vi "Enable_disable State on Multiple Controls.vi"(8 "error in (no error)":errorcluster, 9 "Disabled":T1(ring)=enum."Disabled and Grayed Out", 10 "Disable control?":bool, 11 "Controls":refnum<vi>[](array[refnum])) -> (0 "error out":errorcluster)   [LabVIEW 2014]
doc: "Sets all the controls in the input array to the \"Enable state\" value."
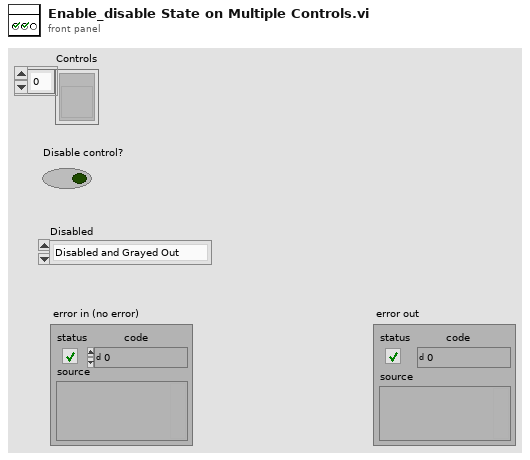
[diagram p1: front panel]
types:
  T1 = enum8{"Enabled", "Disabled", "Disabled and Grayed Out"}
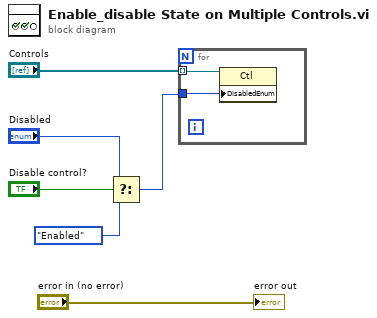
[diagram p0: block diagram]
diagram:
  n1 = Select(t="Disabled", s="Disable control?", f=T1."Enabled" ("Disabled")) -> (s? t:f=w4:T1)
  n2 = for {
    tunnel: "Controls" -> [w8] mode=indexing
    tunnel: w4 -> [w7]
    n3 = property class="Ctl"(reference=w8, "DisabledEnum"=w7) -> ()  [unwired: 1 in, 2 out]
  }
  "error out" <- "error in (no error)"
